vi "CalcCMR Persona.vi"(8 "Zero?":bool, 10 "Ref Sensor 2":dbl, 11 "Ref Sensor":dbl) -> (3 "delta SNS":dbl)   [LabVIEW 2015]
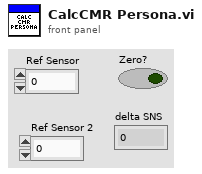
[diagram p1: front panel]
types:
  T1 = cluster{"SNS":dbl, "delta SNS":dbl, "zero SNS":dbl}
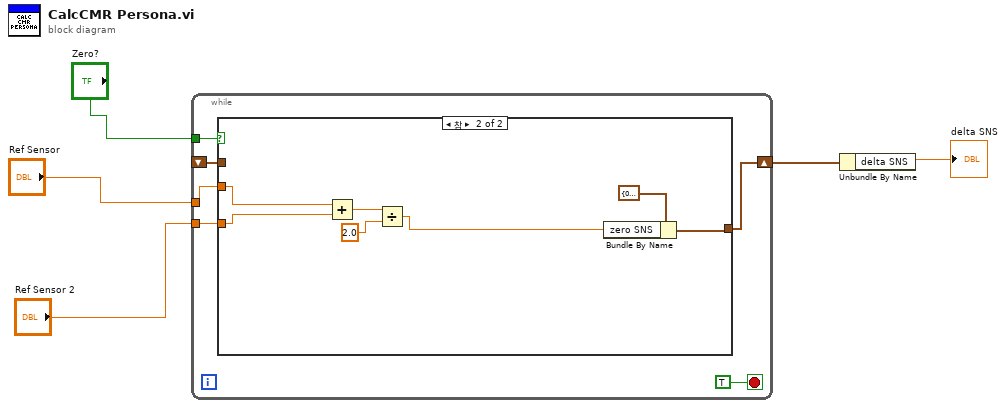
[diagram p0: block diagram]
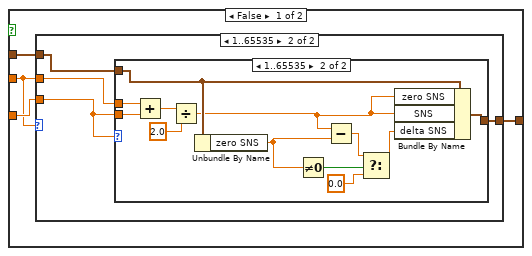
[diagram p2: hidden frame]
diagram:
  n1 = while {
    tunnel: "Ref Sensor 2" -> [w10]
    tunnel: "Ref Sensor" -> [w9]
    tunnel: "Zero?" -> [w8]
    shift-right: [w11] -> w4
    shift-left: _ -> [w7]
    stop <- TRUE stop-if-true
    n2 = case shown="참" w8 {
      tunnel: [w15 w40] -> w11
      tunnel: w7 -> [w14 _]
      tunnel: w10 -> [w13 w34]
      tunnel: w9 -> [w12 w39]
      frame False {
        n3 = case shown="1..65535" w12 {
          tunnel: w12 -> [_ w20]
          tunnel: w13 -> [_ w17]
          tunnel: [w16 w19] -> w15
          tunnel: w14 -> [w16 w18]
          frame 0, Default {
          }
          frame 1..65535 {
            n4 = case shown="1..65535" w17 {
              tunnel: w17 -> [_ w32]
              tunnel: w20 -> [_ w30]
              tunnel: [w21 w29] -> w19
              tunnel: w18 -> [w21 w28]
              frame 0, Default {
              }
              frame 1..65535 {
                n5 = Add(x=w30, y=w32) -> (x+y=w33:dbl)
                n6 = Divide(x=w33, y=2.0) -> (x/y=w27:dbl)
                n7 = Unbundle By Name(w28) -> ("zero SNS"=w26:dbl)
                n8 = Not Equal To 0?(x=w26) -> (x != 0?=w25:bool)
                n9 = Subtract(x=w27, y=w26) -> (x-y=w24:dbl)
                n10 = Select(t=w24, s=w25, f=0.0) -> (s? t:f=w23:dbl)
                n11 = Bundle By Name(cluster=w28, "zero SNS"=w27, "SNS"=w27, "delta SNS"=w23) -> (w29:T1)
              }
            }
          }
        }
      }
      frame True {
        n12 = Add(x=w39, y=w34) -> (x+y=w38:dbl)
        n13 = Divide(x=w38, y=2.0) -> (x/y=w36:dbl)
        n14 = Bundle By Name(cluster=T1 {"SNS"=0.0, "delta SNS"=0.0, "zero SNS"=0.0} ("SNS"), "zero SNS"=w36) -> (w40:T1)
      }
    }
  }
  n15 = Unbundle By Name(w4) -> ("delta SNS"=→"delta SNS":dbl)
